vi "Read zmax.vi"(8 "error in (no error)":errorcluster, 11 "Cube in":refnum<class "Cube.lvclass">) -> (0 "error out":errorcluster, 2 "zmax":i64, 3 "Cube out":refnum<class "Cube.lvclass">)   [LabVIEW 2019, in "22.lvlib" / "Cube.lvclass"]
uses:
  Cube.lvclass
  Cube.lvclass/Cube.ctl
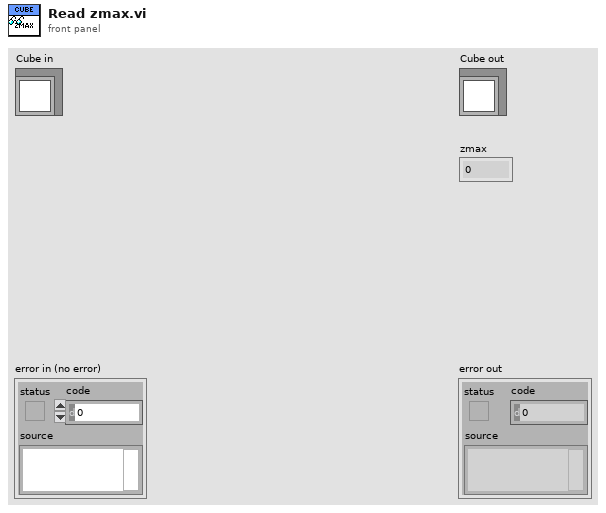
[diagram p1: front panel]
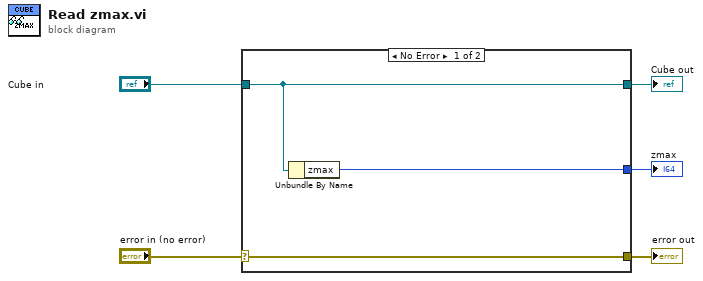
[diagram p0: block diagram]
diagram:
  n1 = case shown="No Error" "error in (no error)" {
    selector: "error in (no error)" -> [w8 w9]
    tunnel: [w8 w9] -> w4
    tunnel: [w7 w10] -> w2
    tunnel: "Cube in" -> [w7 w10]
    tunnel: [w6 _] -> w1
    frame No Error {
      n2 = Unbundle By Name(w7) -> ("zmax"=w6:i64)
    }
    frame Error {
    }
  }
  "error out" <- w4
  "Cube out" <- w2
  "zmax" <- w1
